vi "Generate Table Regular Functions.vi"(8 "Error in":errorcluster, 9 "Table Name":string, 10 "Folder to Saved File":path, 11 "Connection in":refnum<class "Connection.lvclass">) -> (0 "Error out":errorcluster, 2 "SQL-LV File Paths":T1, 3 "Connection out":refnum<class "Connection.lvclass">)   [LabVIEW 2021]
uses:
  <vilib>/drjdpowell/SQLite Library/SQL Connection/Connection.lvclass
  SQL-LV Table File Paths.ctl
  SQL-LV Table Control Paths.ctl
  SQL-LV Table VI Paths.ctl
  edt.lib/sqlite.lib/SQLite Field Info.ctl
  edt.lib/sqlite.lib/SQLite Data Type.ctl
  Field Info to Cluster Item Info (Array).vi
  edt.lib/vie.lib/EDT VIE.lvlib
  edt.lib/sqlite.lib/EDT SQLite+.lvlib
  edt.lib/vi_script.lib/EDT VI Script.lvlib
panel:
  in  "Tab Control":enum32{"Main", "Misc"}(tab)
  out "itr":i32
  out "Previous State":string
  out "Current State":string
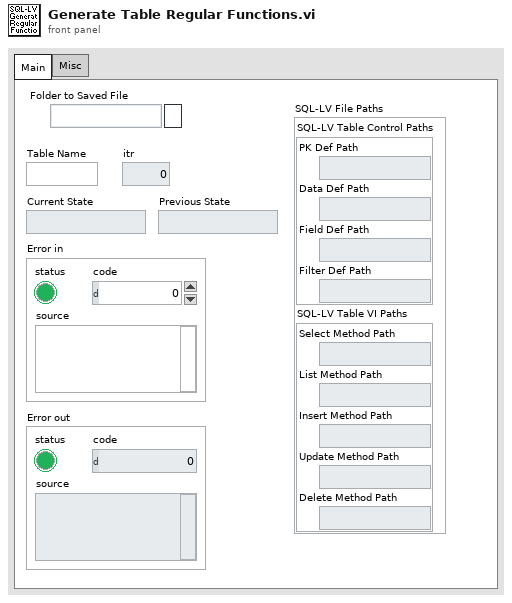
[diagram p1: front panel]
types:
  T1 = typedef "SQL-LV Table File Paths.ctl" = cluster{"SQL-LV Table Control Paths":T2, "SQL-LV Table VI Paths":T3}
  T2 = typedef "SQL-LV Table Control Paths.ctl" = cluster{"PK Def Path":path, "Data Def Path":path, "Field Def Path":path, "Filter Def Path":path}
  T3 = typedef "SQL-LV Table VI Paths.ctl" = cluster{"Select Method Path":path, "List Method Path":path, "Insert Method Path":path, "Update Method Path":path, "Delete Method Path":path}
  T4 = typedef "EDT SQLite+.lvlib/SQLite Field Info.ctl" = cluster{"cid":i32, "name":string, "type":T5, "notnull":bool, "dflt_value":variant, "pk":bool}
  T5 = typedef "EDT SQLite+.lvlib/SQLite Data Type.ctl" = enum16{"INT", "INTEGER", "TINYINT", "SMALLINT", "MEDIUMINT", "BIGINT", "UNSIGNED BIG INT", "INT2", "INT8", "CHARACTER", "VARCHAR", "VARYING CHARACTER", "NCHAR", "NATIVE CHARACTER", "NVARCHAR", "TEXT", "CLOB", "BLOB", "no datatype specified", "REAL", "DOUBLE", "DOUBLE PRECISION", "FLOAT", "NUMERIC", "DECIMAL", "BOOLEAN", "DATE", "DATETIME"}
  T6 = cluster{"Connection in":refnum<class "Connection.lvclass">, "Folder to Saved File":path, "Table Name":string, "SQL-LV File Paths":T1, "Fields Info":T4[]}
  T7 = typedef "EDT VI Script.lvlib/Cluster Item Info.ctl" = cluster{"Label.Text":string, "Type":T8, "Default Value":variant, "Description":string}
  T8 = typedef "NI_Data Type.lvlib/Data Type.ctl" = enum8{"Invalid Type", "Void", "I8", "I16", "I32", "I64", "U8", "U16", "U32", "U64", "Single Float", "Double Float", "Extended Float", "Single Complex", "Double Complex", "Extended Complex", "Enum U8", "Enum U16", "Enum U32", "Enum U64", "Single Float With Unit", "Double Float With Unit", "Extended Float With Unit", "Single Complex with Unit", "Double Complex with Unit", "Extended Complex with Unit", "Boolean", "String", "Path", "Picture", "Tag", "Array", "Cluster", "Variant", "LV Variant", "Waveform", "Timestamp", "Digital Waveform", "Digital Data", "ExpressData", "Refnum", "External Data", "VI", "Poly VI", "LabVIEW Class Instance", "Fixed Point", "Set Collection", "Map Collection"}
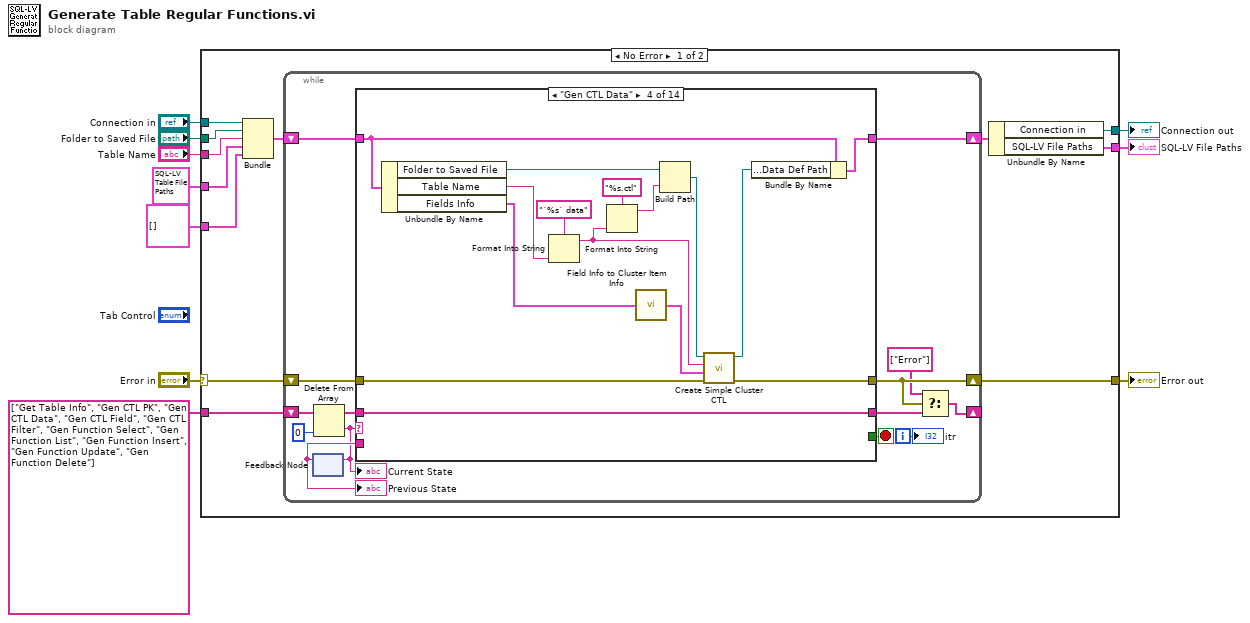
[diagram p0: block diagram]
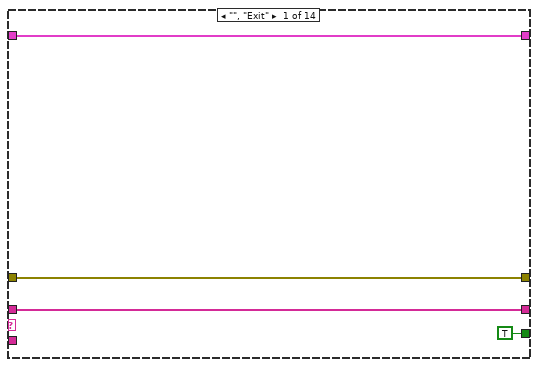
[diagram p2: hidden frame]
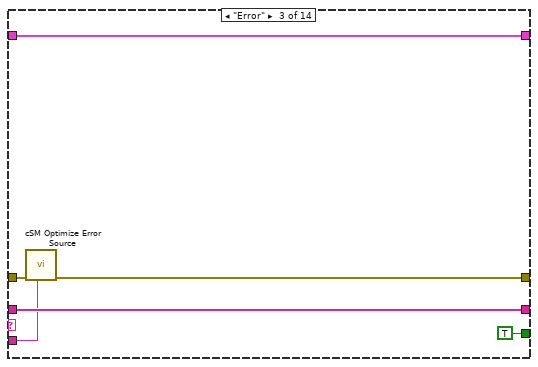
[diagram p4: hidden frame]
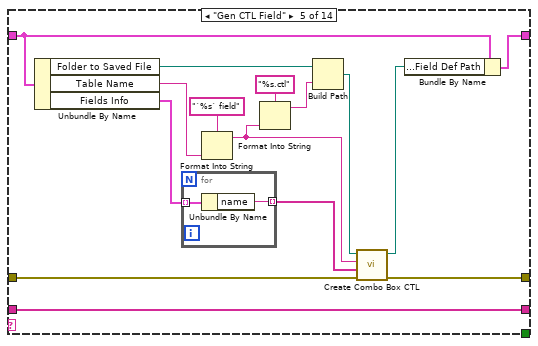
[diagram p5: hidden frame]
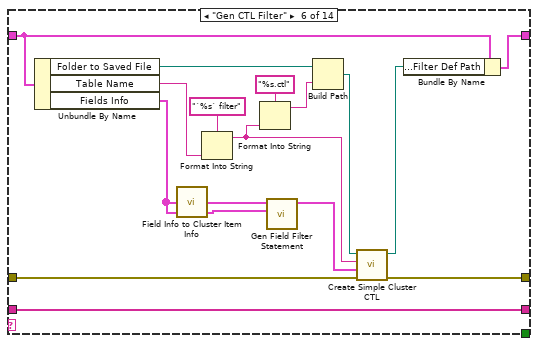
[diagram p6: hidden frame]
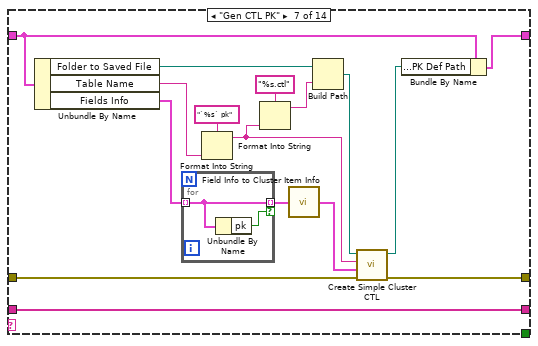
[diagram p7: hidden frame]
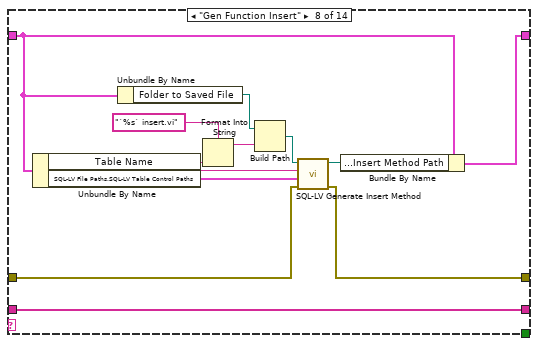
[diagram p8: hidden frame]
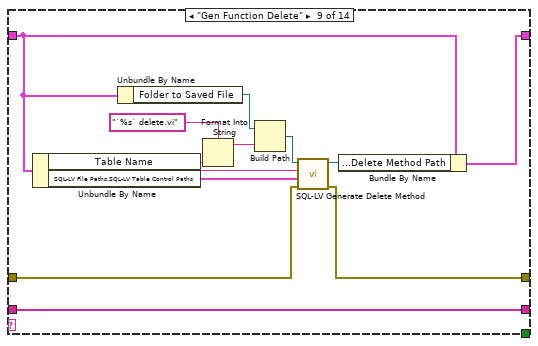
[diagram p9: hidden frame]
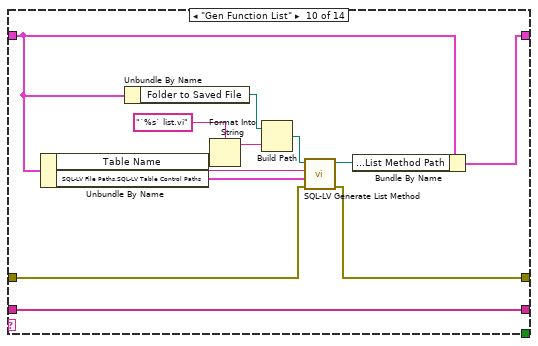
[diagram p10: hidden frame]
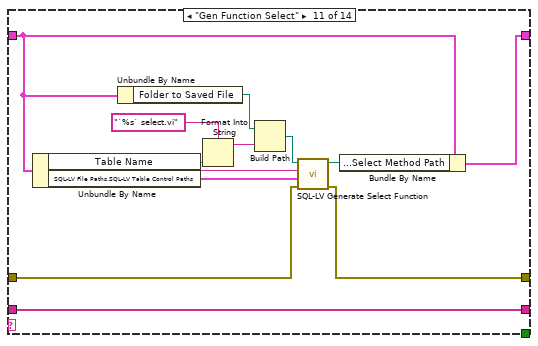
[diagram p11: hidden frame]
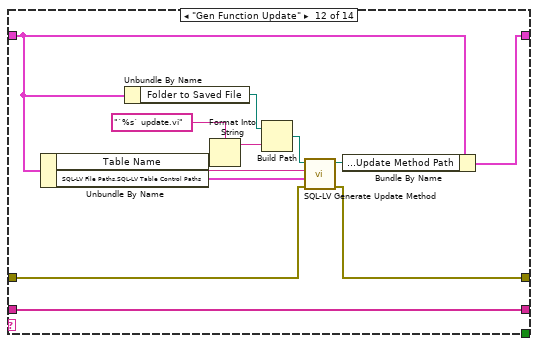
[diagram p12: hidden frame]
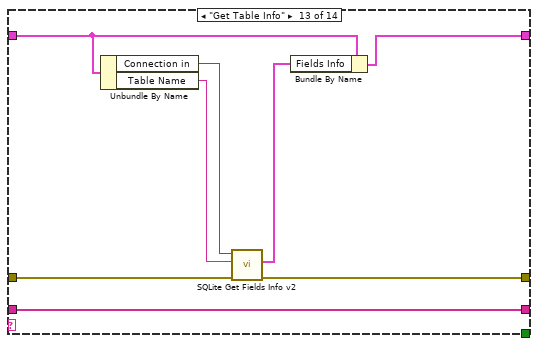
[diagram p13: hidden frame]
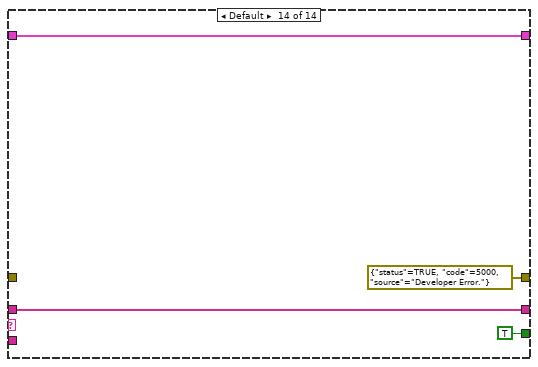
[diagram p14: hidden frame]
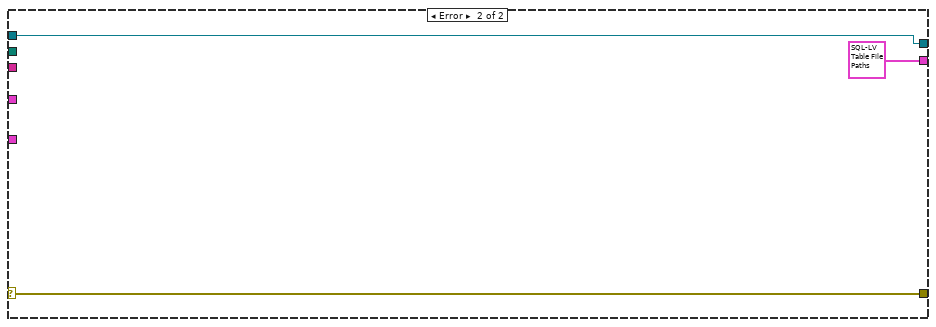
[diagram p15: hidden frame]
diagram:
  n1 = case shown="No Error" "Error in" {
    selector: "Error in" -> [w20 w190]
    tunnel: string[] ["Get Table Info", "Gen CTL PK", "Gen CTL Data", "Gen CTL Field", "Gen CTL Filter", "Gen Function Select", "Gen Function List", "Gen Function Insert", "Gen Function Update", "Gen Function Delete"] ("Initial States") -> [w22 _]
    tunnel: [w21 w190] -> w8
    tunnel: "Folder to Saved File" -> [w19 _]
    tunnel: "Table Name" -> [w18 _]
    tunnel: T1 {"SQL-LV Table Control Paths"={"PK Def Path"=path "", "Data Def Path"=path "", "Field Def Path"=path "", "Filter Def Path"=path ""}, "SQL-LV Table VI Paths"={"Select Method Path"=path "", "List Method Path"=path "", "Insert Method Path"=path "", "Update Method Path"=path "", "Delete Method Path"=path ""}} ("SQL-LV File Paths") -> [w16 _]
    tunnel: [w14 T1 {"SQL-LV Table Control Paths"={"PK Def Path"=path "", "Data Def Path"=path "", "Field Def Path"=path "", "Filter Def Path"=path ""}, "SQL-LV Table VI Paths"={"Select Method Path"=path "", "List Method Path"=path "", "Insert Method Path"=path "", "Update Method Path"=path "", "Delete Method Path"=path ""}} ("SQL-LV File Paths")] -> w4
    tunnel: T4[] [] ("Fields Info") -> [w13 _]
    tunnel: "Connection in" -> [w12 w188]
    tunnel: [w11 w188] -> w1
    frame No Error {
      n2 = Bundle("Connection in"=w12, "Folder to Saved File"=w19, "Table Name"=w18, "SQL-LV File Paths"=w16, "Fields Info"=w13) -> (w17:T6)  [unwired: 1 in]
      n3 = while {
        shift-right: [w30] -> _
        shift-left: w22 -> [w36]
        shift-right: [w29] -> w21
        shift-left: w20 -> [w33]
        shift-right: [w25] -> w15
        shift-left: w17 -> [w26]
        i -> [w34]
        stop <- w32 stop-if-true
        n4 = feedback #1() -> (w28:string)  [unwired: 1 in]
        "Previous State" <- w28
        n5 = Delete From Array(array=w36, index=0) -> (deleted portion=w27:string, array with subset deleted=w35:string[])  [unwired: 1 in]
        "Current State" <- w27
        n6 = feedback-in #1(w27) -> ()
        n7 = case shown="\"Gen CTL Data\"" w27 {
          tunnel: [w40 w43 w49 w64 w79 w97 w113 w127 w139 w151 w163 w175 w183 w185] -> w31
          tunnel: w35 -> [w40 w43 w49 w64 w79 w97 w113 w127 w139 w151 w163 w175 w183 w185]
          tunnel: w33 -> [w39 w42 w47 w56 w72 w91 w104 w122 w134 w146 w158 w170 w182 _]
          tunnel: [w39 w42 w46 w50 w65 w82 w98 w121 w133 w145 w157 w169 w180 errorcluster {"status"=TRUE, "code"=5000, "source"="Developer Error."} ("error in")] -> w29
          tunnel: [TRUE _ TRUE _ _ _ _ _ _ _ _ _ _ TRUE] -> w32
          tunnel: w28 -> [_ _ w45 _ _ _ _ _ _ _ _ _ _ _]
          tunnel: w26 -> [w37 w41 w44 w63 w78 w96 w112 w120 w132 w144 w156 w168 w179 w184]
          tunnel: [w37 w41 w44 w52 w68 w87 w100 w119 w131 w143 w155 w167 w178 w184] -> w25
          frame "", "Exit" {
          }
          frame "<<KEEP>>" {
          }
          frame "Error" {
            n8 = call "cSM Optimize Error Source.vi"("Previous State"=w45, "Error in"=w47) -> ("Error out"=w46:errorcluster)  [unwired: 9 in]
          }
          frame "Gen CTL Data" {
            n9 = Unbundle By Name(w63) -> ("Folder to Saved File"=w54:path, "Table Name"=w59:string, "Fields Info"=w60:T4[])
            n10 = Format Into String(format string="`%s` data", w59) -> (resulting string=w57:string)  [unwired: 2 in, 1 out]
            n11 = Format Into String(format string="%s.ctl", w57) -> (resulting string=w55:string)  [unwired: 2 in, 1 out]
            n12 = call-poly "Field Info to Cluster Item Info.vi"("Fields Info"=w60) -> ("Cluster Items"=w61:T7[])
            n13 = Build Path(base path=w54, name or relative path=w55) -> (appended path=w53:path)
            n14 = call "Create Simple Cluster CTL.vi"("error in (no error)"=w56, "Cluster Item"=w61, "Label Name"=w57, "File Save Path"=w53) -> ("error out"=w50:errorcluster, "Path"=w51:path)  [unwired: 6 in]
            n15 = Bundle By Name(cluster=w63, "SQL-LV File Paths.SQL-LV Table Control Paths.Data Def Path"=w51) -> (w52:T6)
          }
          frame "Gen CTL Field" {
            n16 = Unbundle By Name(w78) -> ("Folder to Saved File"=w70:path, "Table Name"=w75:string, "Fields Info"=w76:T4[])
            n17 = for {
              tunnel: w76 -> [w81] mode=indexing
              tunnel: [w80] -> w66 mode=indexing
              n18 = Unbundle By Name(w81) -> ("name"=w80:string)
            }
            n19 = Format Into String(format string="`%s` field", w75) -> (resulting string=w73:string)  [unwired: 2 in, 1 out]
            n20 = Format Into String(format string="%s.ctl", w73) -> (resulting string=w71:string)  [unwired: 2 in, 1 out]
            n21 = Build Path(base path=w70, name or relative path=w71) -> (appended path=w69:path)
            n22 = call "Create Combo Box CTL.vi"("error in (no error)"=w72, "Items"=w66, "Label Name"=w73, "Folder to Saved File"=w69) -> ("error out"=w65:errorcluster, "Path"=w67:path)  [unwired: 6 in]
            n23 = Bundle By Name(cluster=w78, "SQL-LV File Paths.SQL-LV Table Control Paths.Field Def Path"=w67) -> (w68:T6)
          }
          frame "Gen CTL Filter" {
            n24 = Unbundle By Name(w96) -> ("Folder to Saved File"=w89:path, "Table Name"=w94:string, "Fields Info"=w83:T4[])
            n25 = call-poly "Field Info to Cluster Item Info.vi"("Fields Info"=w83) -> ("Cluster Items"=w85:T7[])
            n26 = Format Into String(format string="`%s` filter", w94) -> (resulting string=w92:string)  [unwired: 2 in, 1 out]
            n27 = Format Into String(format string="%s.ctl", w92) -> (resulting string=w90:string)  [unwired: 2 in, 1 out]
            n28 = call "Gen Field Filter Statement.vi"("Fields Info"=w83, "Cluster Items in"=w85) -> ("Cluster Items out"=w84:T7[])  [unwired: 9 in]
            n29 = Build Path(base path=w89, name or relative path=w90) -> (appended path=w88:path)
            n30 = call "Create Simple Cluster CTL.vi"("error in (no error)"=w91, "Cluster Item"=w84, "Label Name"=w92, "File Save Path"=w88) -> ("error out"=w82:errorcluster, "Path"=w86:path)  [unwired: 6 in]
            n31 = Bundle By Name(cluster=w96, "SQL-LV File Paths.SQL-LV Table Control Paths.Filter Def Path"=w86) -> (w87:T6)
          }
          frame "Gen CTL PK" {
            n32 = Unbundle By Name(w112) -> ("Folder to Saved File"=w102:path, "Table Name"=w107:string, "Fields Info"=w108:T4[])
            n33 = for {
              tunnel: w108 -> [w115] mode=indexing
              tunnel: [w115] -> w111 mode=indexing if=w114
              n34 = Unbundle By Name(w115) -> ("pk"=w114:bool)
            }
            n35 = Format Into String(format string="`%s` pk", w107) -> (resulting string=w105:string)  [unwired: 2 in, 1 out]
            n36 = Format Into String(format string="%s.ctl", w105) -> (resulting string=w103:string)  [unwired: 2 in, 1 out]
            n37 = call-poly "Field Info to Cluster Item Info.vi"("Fields Info"=w111) -> ("Cluster Items"=w109:T7[])
            n38 = Build Path(base path=w102, name or relative path=w103) -> (appended path=w101:path)
            n39 = call "Create Simple Cluster CTL.vi"("error in (no error)"=w104, "Cluster Item"=w109, "Label Name"=w105, "File Save Path"=w101) -> ("error out"=w98:errorcluster, "Path"=w99:path)  [unwired: 6 in]
            n40 = Bundle By Name(cluster=w112, "SQL-LV File Paths.SQL-LV Table Control Paths.PK Def Path"=w99) -> (w100:T6)
          }
          frame "Gen Function Insert" {
            n41 = Unbundle By Name(w120) -> ("Table Name"=w117:string, "SQL-LV File Paths.SQL-LV Table Control Paths"=w116:T2)
            n42 = Unbundle By Name(w120) -> ("Folder to Saved File"=w125:path)
            n43 = Format Into String(format string="`%s` insert.vi", w117) -> (resulting string=w124:string)  [unwired: 2 in, 1 out]
            n44 = Build Path(base path=w125, name or relative path=w124) -> (appended path=w123:path)
            n45 = call "SQL-LV Generate Insert Method.vi"("error in (no error)"=w122, "SQL-LV Control Paths"=w116, "Table Name"=w117, "Save as"=w123) -> ("error out"=w121:errorcluster, "Save as out"=w118:path)  [unwired: 6 in]
            n46 = Bundle By Name(cluster=w120, "SQL-LV File Paths.SQL-LV Table VI Paths.Insert Method Path"=w118) -> (w119:T6)
          }
          frame "Gen Function Delete" {
            n47 = Unbundle By Name(w132) -> ("Table Name"=w129:string, "SQL-LV File Paths.SQL-LV Table Control Paths"=w128:T2)
            n48 = Unbundle By Name(w132) -> ("Folder to Saved File"=w137:path)
            n49 = Format Into String(format string="`%s` delete.vi", w129) -> (resulting string=w136:string)  [unwired: 2 in, 1 out]
            n50 = Build Path(base path=w137, name or relative path=w136) -> (appended path=w135:path)
            n51 = call "SQL-LV Generate Delete Method.vi"("error in (no error)"=w134, "SQL-LV Control Paths"=w128, "Table Name"=w129, "Save as"=w135) -> ("error out"=w133:errorcluster, "Save as out"=w130:path)  [unwired: 6 in]
            n52 = Bundle By Name(cluster=w132, "SQL-LV File Paths.SQL-LV Table VI Paths.Delete Method Path"=w130) -> (w131:T6)
          }
          frame "Gen Function List" {
            n53 = Unbundle By Name(w144) -> ("Table Name"=w141:string, "SQL-LV File Paths.SQL-LV Table Control Paths"=w140:T2)
            n54 = Unbundle By Name(w144) -> ("Folder to Saved File"=w149:path)
            n55 = Format Into String(format string="`%s` list.vi", w141) -> (resulting string=w148:string)  [unwired: 2 in, 1 out]
            n56 = Build Path(base path=w149, name or relative path=w148) -> (appended path=w147:path)
            n57 = call "SQL-LV Generate List Method.vi"("error in (no error)"=w146, "SQL-LV Control Paths"=w140, "Table Name"=w141, "Save as"=w147) -> ("error out"=w145:errorcluster, "Save as out"=w142:path)  [unwired: 6 in]
            n58 = Bundle By Name(cluster=w144, "SQL-LV File Paths.SQL-LV Table VI Paths.List Method Path"=w142) -> (w143:T6)
          }
          frame "Gen Function Select" {
            n59 = Unbundle By Name(w156) -> ("Table Name"=w153:string, "SQL-LV File Paths.SQL-LV Table Control Paths"=w152:T2)
            n60 = Unbundle By Name(w156) -> ("Folder to Saved File"=w161:path)
            n61 = Format Into String(format string="`%s` select.vi", w153) -> (resulting string=w160:string)  [unwired: 2 in, 1 out]
            n62 = Build Path(base path=w161, name or relative path=w160) -> (appended path=w159:path)
            n63 = call "SQL-LV Generate Select Function.vi"("error in (no error)"=w158, "SQL-LV File Paths.SQL-LV Control Paths"=w152, "Table Name"=w153, "Save as"=w159) -> ("error out"=w157:errorcluster, "Save as out"=w154:path)  [unwired: 6 in]
            n64 = Bundle By Name(cluster=w156, "SQL-LV File Paths.SQL-LV Table VI Paths.Select Method Path"=w154) -> (w155:T6)
          }
          frame "Gen Function Update" {
            n65 = Unbundle By Name(w168) -> ("Table Name"=w165:string, "SQL-LV File Paths.SQL-LV Table Control Paths"=w164:T2)
            n66 = Unbundle By Name(w168) -> ("Folder to Saved File"=w173:path)
            n67 = Format Into String(format string="`%s` update.vi", w165) -> (resulting string=w172:string)  [unwired: 2 in, 1 out]
            n68 = Build Path(base path=w173, name or relative path=w172) -> (appended path=w171:path)
            n69 = call "SQL-LV Generate Update Method.vi"("error in (no error)"=w170, "SQL-LV Control Paths"=w164, "Table Name"=w165, "Save as"=w171) -> ("error out"=w169:errorcluster, "Save as out"=w166:path)  [unwired: 6 in]
            n70 = Bundle By Name(cluster=w168, "SQL-LV File Paths.SQL-LV Table VI Paths.Update Method Path"=w166) -> (w167:T6)
          }
          frame "Get Table Info" {
            n71 = Unbundle By Name(w179) -> ("Connection in"=w176:refnum<class "Connection.lvclass">, "Table Name"=w181:string)
            n72 = call "SQLite Get Fields Info v2.vi"("error in"=w182, "Table Name"=w181, "SQLite Connection"=w176) -> ("error out"=w180:errorcluster, "Fields Info"=w177:T4[])  [unwired: 6 in, 1 out]
            n73 = Bundle By Name(cluster=w179, "Fields Info"=w177) -> (w178:T6)
          }
          frame Default {
          }
        }
        n74 = Select(t=string[] ["Error"], s=w29, f=w31) -> (s? t:f=w30:string[])
        "itr" <- w34
      }
      n75 = Unbundle By Name(w15) -> ("Connection in"=w11:refnum<class "Connection.lvclass">, "SQL-LV File Paths"=w14:T1)
    }
    frame Error {
    }
  }
  "Error out" <- w8
  "Connection out" <- w1
  "SQL-LV File Paths" <- w4
